vi "U32ToSGL.vi"(11 "U32":u32) -> (3 "SGL":sgl format="%#.6f")   [LabVIEW 2016]
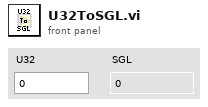
[diagram p1: front panel]
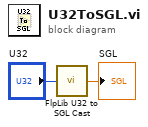
[diagram p0: block diagram]
diagram:
  n1 = call <userlib>:"FlpLib U32 to SGL Cast.vi"("x"="U32") -> ("y"=→"SGL":sgl)  [unwired: 4 in]
